vi "Get and Set Control Description and Strip.vi"(8 "错误输入（无错误）":errorcluster, 9 "Mode":enum16{"Read", "Write"}(ring), 10 "Info In":cluster{"说明信息":string, "提示框":string}, 11 "Ctl Ref In":refnum<vi>) -> (0 "错误输出":errorcluster, 2 "Info Out":cluster{"说明信息":string, "提示框":string}, 3 "Ctl Ref Out":refnum<vi>)   [LabVIEW 2012, in "CtrlRef.lvlib"]
uses:
  CtrlRef.lvlib
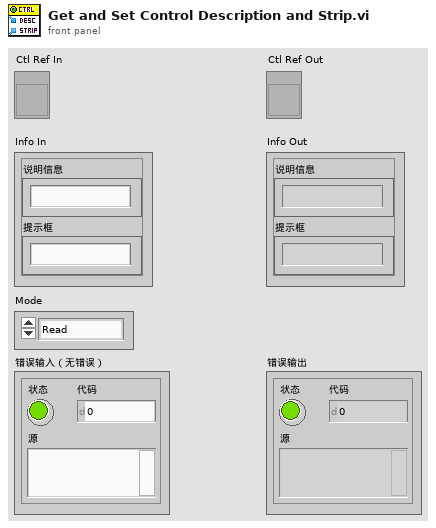
[diagram p1: front panel]
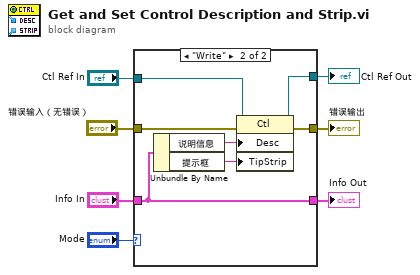
[diagram p0: block diagram]
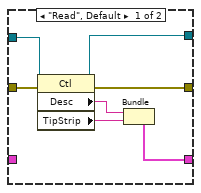
[diagram p2: hidden frame]
diagram:
  n1 = case shown="\"Write\"" "Mode" {
    tunnel: "错误输入（无错误）" -> [w14 w20]
    tunnel: [w13 w18] -> w5
    tunnel: "Ctl Ref In" -> [w12 w21]
    tunnel: [w11 w19] -> w3
    tunnel: [w8 w15] -> w2
    tunnel: "Info In" -> [_ w15]
    frame "Read", Default {
      n2 = property class="Ctl"(reference=w12, error in=w14) -> (reference out=w11:refnum<vi>, error out=w13:errorcluster, "Desc"=w10:string, "TipStrip"=w9:string)
      n3 = Bundle("Desc"=w10, "TipStrip"=w9) -> (w8:cluster{"Desc":string, "TipStrip":string})  [unwired: 1 in]
    }
    frame "Write" {
      n4 = Unbundle By Name(w15) -> ("说明信息"=w17:string, "提示框"=w16:string)
      n5 = property class="Ctl"(reference=w21, error in=w20, "Desc"=w17, "TipStrip"=w16) -> (reference out=w19:refnum<vi>, error out=w18:errorcluster)
    }
  }
  "错误输出" <- w5
  "Ctl Ref Out" <- w3
  "Info Out" <- w2
